vi "subVI_temp.vi"(11 "VISA Refnum in":refnum<visa-resource-name>) -> (0 "error out":errorcluster, 2 "Unit Address (1)":u8, 3 "VISA Refnum out":refnum<visa-resource-name>)   [LabVIEW 2013]
uses:
  <instrlib>/Eurotherm 32xx Series/Eurotherm 32xx Series.lvlib
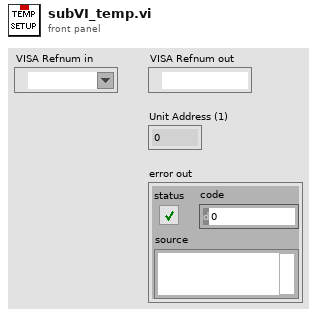
[diagram p1: front panel]
types:
  T1 = cluster{"Baud Rate (19200)":u32, "Parity (0: None)":u16, "Break Length (0)":u16}
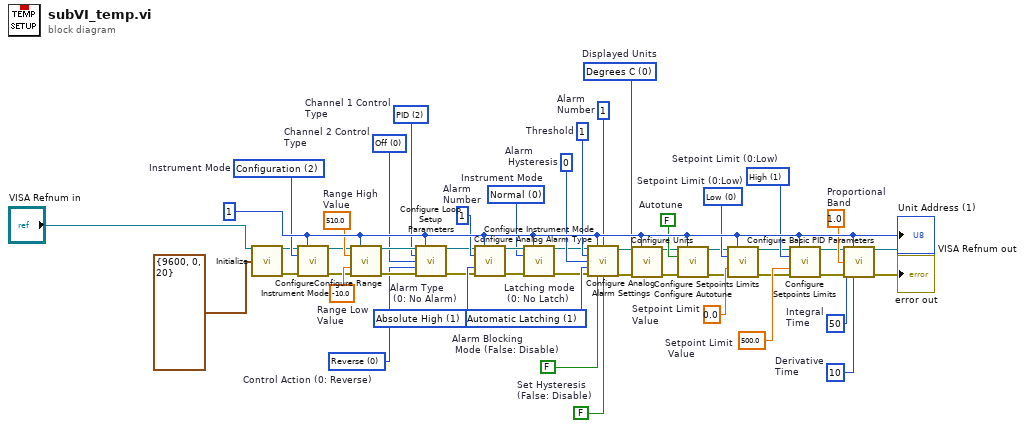
[diagram p0: block diagram]
diagram:
  w51 = u8 1 ("Unit Address (1)")
  w47 = sgl 500.0  # Setpoint Limit  Value
  w44 = sgl -10.0  # Range Low  Value
  w43 = sgl 510.0  # Range High Value
  w42 = u16 0 items=["Reverse", "Direct"]  # Control Action (0: Reverse)
  w41 = u16 0 items=["Low", "High"]  # Setpoint Limit (0:Low)
  w40 = u16 1 items=["Low", "High"]  # Setpoint Limit (0:Low)
  w37 = FALSE  # Set Hysteresis  (False: Disable)
  w29 = 10  # Derivative  Time
  w28 = 50  # Integral  Time
  w27 = sgl 1.0  # Proportional  Band
  w26 = sgl 0.0  # Setpoint Limit  Value
  w19 = FALSE  # Autotune
  w18 = u8 0 items=[" Degrees C", " Degrees F", " Degrees K"]  # Displayed Units
  w36 = FALSE  # Alarm Blocking  Mode (False: Disable)
  w35 = u16 1 items=["No Latch", "Automatic Latching", "Manual Latching", "Event Latching"]  # Latching mode  (0: No Latch)
  w34 = u16 0  # Alarm  Hysteresis
  w33 = u16 1  # Threshold
  w32 = u16 1  # Alarm  Number
  w13 = u8 1 items=["No Alarm", "Absolute High", "Absolute Low", "Deviation High", "Deviation Low", "Deviation Band", "Rising Rate of Change Alarm", "Falling Rate of Change Alarm"]  # Alarm Type  (0: No Alarm)
  w12 = u16 1  # Alarm  Number
  w7 = u8 0 items=["Normal", "StandBy", "Configuration"]  # Instrument Mode
  w6 = u8 0 items=["Off", "On/Off", "PID", "VPU", "VPB"]  # Channel 2 Control  Type
  w5 = u8 2 items=["Off", "On/Off", "PID", "VPU", "VPB"]  # Channel 1 Control  Type
  w2 = u8 2 items=["Normal", "StandBy", "Configuration"]  # Instrument Mode
  n1 = call <instrlib>:"Initialize.vi"("VISA resource name"="VISA Refnum in", "Serial Configuration"=T1 {"Baud Rate (19200)"=9600, "Parity (0: None)"=0, "Break Length (0)"=20}) -> ("VISA resource name out"=w1:refnum<visa-resource-name>, "error out"=w48:errorcluster)  [unwired: 12 in]
  n2 = call <instrlib>:"Configure Instrument Mode.vi"("VISA resource name"=w1, "Unit Address (1)"=w51, "Instrument Mode (0: Normal)"=w2, "error in (no error)"=w48) -> ("VISA resource name out"=w3:refnum<visa-resource-name>, "error out"=w4:errorcluster)  [unwired: 10 in]
  n3 = call <instrlib>:"Configure Range.vi"("VISA resource name"=w3, "Unit Address (1)"=w51, "Range High (0)"=w43, "Range Low (0)"=w44, "error in (no error)"=w4) -> ("VISA resource name out"=w45:refnum<visa-resource-name>, "error out"=w46:errorcluster)  [unwired: 9 in]
  n4 = call <instrlib>:"Configure Loop Setup Parameters.vi"("VISA resource name"=w45, "Unit Address (1)"=w51, "Channel 1 Control Algorithm (0: Off)"=w5, "Channel 2 Control Algorithm (0: Off)"=w6, "Control Action (0: Reverse)"=w42, "error in (no error)"=w46) -> ("VISA resource name out"=w8:refnum<visa-resource-name>, "error out"=w9:errorcluster)  [unwired: 8 in]
  n5 = call <instrlib>:"Configure Analog Alarm Type.vi"("VISA resource name"=w8, "Unit Address (1)"=w51, "Alarm Number (1)"=w12, "Alarm Type (0: No Alarm)"=w13, "error in (no error)"=w9) -> ("VISA resource name out"=w10:refnum<visa-resource-name>, "error out"=w11:errorcluster)  [unwired: 9 in]
  n6 = call <instrlib>:"Configure Instrument Mode.vi"("VISA resource name"=w10, "Unit Address (1)"=w51, "Instrument Mode (0: Normal)"=w7, "error in (no error)"=w11) -> ("VISA resource name out"=w30:refnum<visa-resource-name>, "error out"=w31:errorcluster)  [unwired: 10 in]
  n7 = call <instrlib>:"Configure Analog Alarm Settings.vi"("VISA resource name"=w30, "Unit Address (1)"=w51, "Alarm Number (1)"=w32, "Threshold (0)"=w33, "Alarm Hysteresis (1)"=w34, "Latching Mode (0: No Latch)"=w35, "error in (no error)"=w31, "Enable Alarm Blocking (False: Disable)"=w36, "Enable Hysteresis (False: Disable)"=w37) -> ("VISA resource name out"=w38:refnum<visa-resource-name>, "error out"=w39:errorcluster)  [unwired: 5 in]
  n8 = call <instrlib>:"Configure Units.vi"("VISA resource name"=w38, "Unit Address (1)"=w51, "Displayed Units (0: Degrees C)"=w18, "error in (no error)"=w39) -> ("VISA resource name out"=w14:refnum<visa-resource-name>, "error out"=w15:errorcluster)  [unwired: 10 in]
  n9 = call <instrlib>:"Configure Autotune.vi"("VISA resource name"=w14, "Unit Address (1)"=w51, "Enable Autotune  (False: Disable)"=w19, "error in (no error)"=w15) -> ("VISA resource name out"=w20:refnum<visa-resource-name>, "error out"=w21:errorcluster)  [unwired: 10 in]
  n10 = call <instrlib>:"Configure Setpoints Limits.vi"("VISA resource name"=w20, "Unit Address (1)"=w51, "Setpoint Limit (0:Low)"=w41, "Setpoint Limit Value (0)"=w26, "error in (no error)"=w21) -> ("VISA resource name out"=w16:refnum<visa-resource-name>, "error out"=w17:errorcluster)  [unwired: 9 in]
  n11 = call <instrlib>:"Configure Setpoints Limits.vi"("VISA resource name"=w16, "Unit Address (1)"=w51, "Setpoint Limit (0:Low)"=w40, "Setpoint Limit Value (0)"=w47, "error in (no error)"=w17) -> ("VISA resource name out"=w22:refnum<visa-resource-name>, "error out"=w25:errorcluster)  [unwired: 9 in]
  n12 = call <instrlib>:"Configure Basic PID Parameters.vi"("VISA resource name"=w22, "Unit Address (1)"=w51, "Proportional Band (1)"=w27, "Integral Time (1)"=w28, "error in (no error)"=w25, "Derivative Time (0)"=w29) -> ("VISA resource name out"=→"VISA Refnum out":refnum<visa-resource-name>, "error out"=→"error out":errorcluster)  [unwired: 8 in]
  "Unit Address (1)" <- w51
